vi "Calling a Private .NET Assembly.vi"() -> ()   [LabVIEW 2023]
doc: "Demonstrates how to call a private .NET assembly. The Constructor Node is called to create an instance of a .NET object. Invoke Nodes are then used to call any method that exists in the chosen .NET assembly."
uses:
  c:/dev/_r/4/eng/lv-core/lvpostprocessingd/lv_mc_x86_64/dist_i386/examples/Connectivity/Dot NET/Calculator.dll
  Calculator.dll
panel:
  in  "Operation":u16(ring) items=["Add", "Subtract", "Multiply", "Divide"]
  out "Result":dbl
  in  "Input 2":dbl=4.0
  in  "Input 1":dbl=2.0
  # "Overview: Demonstrates how to call a private .NET assembly.\nRequirements: Windows\nInstructions:\n1. Enter values for Input 1 and Input 2.\n2. Select an Operation to perform on the two values.\n3. Run the VI to see the result of the selected operation."
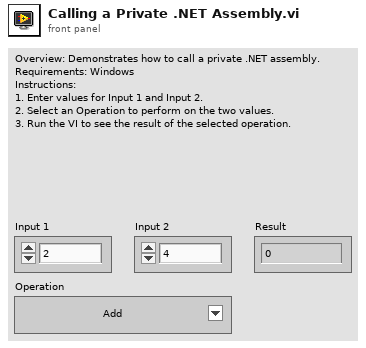
[diagram p1: front panel]
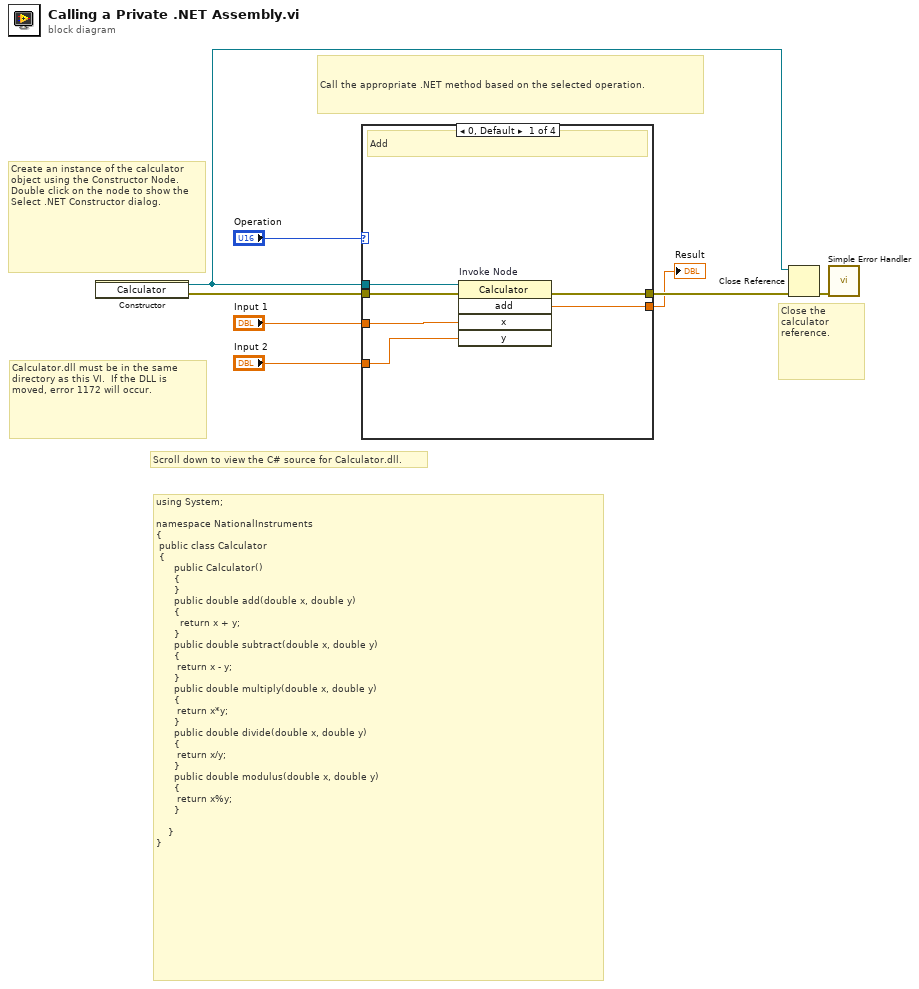
[diagram p0: block diagram]
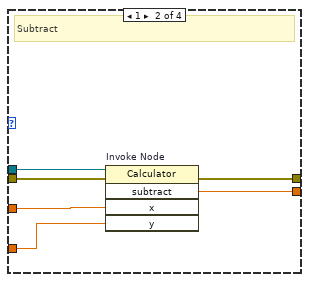
[diagram p2: hidden frame]
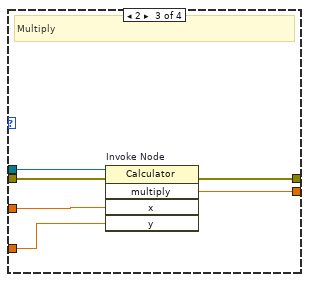
[diagram p3: hidden frame]
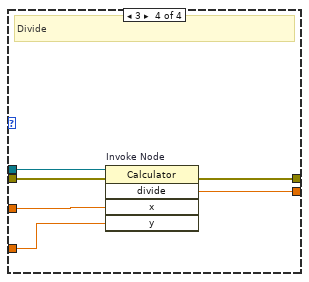
[diagram p4: hidden frame]
diagram:
  # "Call the appropriate .NET method based on the selected operation."
  # "Scroll down to view the C# source for Calculator.dll."
  # "Calculator.dll must be in the same directory as this VI.  If the DLL is moved, error 1172 will occur."
  # "using System;\n\nnamespace NationalInstruments\n{\n\tpublic class Calculator\n\t{\n\t\t    public Calculator()\n\t\t    {\n\t    \t}\n\t\t    public double add(double x, double y)\n\t\t    {\n\t\t\t\t\t   return x + y;\n\t\t\t\t  }\n\t\t    public double subtract(double x, double y)\n\t\t    {\n\t\t\t    return x - y;\n\t\t    }\n\t\t    public double multiply(double x, double y)\n\t\t    {\n\t\t\t    return x*y;\n\t\t    }\n\t\t    public double divide(double x, double y)\n\t\t    {\n\t\t\t    return x/y;\n\t\t    }\n\t\t    public double modulus(double x, double y)\n\t\t    {\n\t\t\t    return x%y;\n\t\t    }\n\t\t\n\t   }\n}"
  # "Close the calculator reference."
  # "Create an instance of the calculator object using the Constructor Node. Double click on the node to show the Select .NET Constructor dialog."
  n1 = constructor class="Calculator"() -> (reference out=w5:refnum<k24>, error out=w6:errorcluster)  [unwired: 3 in, 1 out]
  n2 = case shown="0, Default" "Operation" {
    tunnel: [w14 w20 w26 w32] -> w8
    tunnel: w6 -> [w13 w19 w25 w31]
    tunnel: w5 -> [w12 w18 w24 w30]
    tunnel: [w11 w17 w23 w29] -> w4
    tunnel: "Input 1" -> [w10 w16 w22 w28]
    tunnel: "Input 2" -> [w9 w15 w21 w27]
    frame 0, Default {
      # "Add"
      n3 = invoke on="Invoke Node" class="Calculator" method="add"(reference=w12, error in=w13, "x"=w10, "y"=w9) -> (error out=w14:errorcluster, "add"=w11:dbl)  [unwired: 1 in, 3 out]
    }
    frame 1 {
      # "Subtract"
      n4 = invoke on="Invoke Node" class="Calculator" method="subtract"(reference=w18, error in=w19, "x"=w16, "y"=w15) -> (error out=w20:errorcluster, "subtract"=w17:dbl)  [unwired: 1 in, 3 out]
    }
    frame 2 {
      # "Multiply"
      n5 = invoke on="Invoke Node" class="Calculator" method="multiply"(reference=w24, error in=w25, "x"=w22, "y"=w21) -> (error out=w26:errorcluster, "multiply"=w23:dbl)  [unwired: 1 in, 3 out]
    }
    frame 3 {
      # "Divide"
      n6 = invoke on="Invoke Node" class="Calculator" method="divide"(reference=w30, error in=w31, "x"=w28, "y"=w27) -> (error out=w32:errorcluster, "divide"=w29:dbl)  [unwired: 1 in, 3 out]
    }
  }
  "Result" <- w4
  n7 = Close Reference(reference=w5, error in (no error)=w8) -> (error out=w7:errorcluster)
  n8 = call <vilib>:"Simple Error Handler.vi"("error in (no error)"=w7) -> ()  [unwired: 4 in, 5 out]
